vi "Content.vi"(7 "Context":refnum<class "Context.lvclass">, 8 "Error In":errorcluster, 11 "Comment In":refnum<class "Comment.lvclass">) -> (0 "Error Out":errorcluster, 2 "Content":string, 3 "Comment Out":refnum<class "Comment.lvclass">)   [LabVIEW 2018, in "Toolkit.lvlib" / "Nodes.lvlib" / "Comment.lvclass"]
uses:
  Comment.lvclass
  Support/Context/Context.lvclass
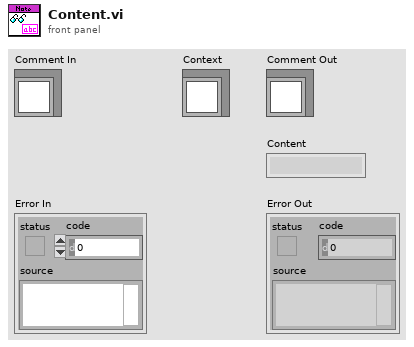
[diagram p1: front panel]
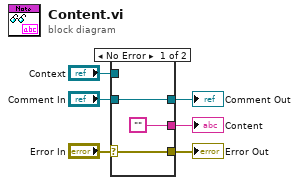
[diagram p0: block diagram]
diagram:
  n1 = case shown="No Error" "Error In" {
    selector: "Error In" -> [w9 w11]
    tunnel: [w9 w11] -> w5
    tunnel: "Comment In" -> [w8 w10]
    tunnel: [w8 w10] -> w2
    tunnel: "Context" -> [_ _]
    tunnel: ["" _] -> w1
    frame No Error {
    }
    frame Error {
    }
  }
  "Error Out" <- w5
  "Content" <- w1
  "Comment Out" <- w2
